vi "bucketOf.vi"(8 "error in (no error)":errorcluster, 10 "Key":string, 11 "HashMap in":refnum<class "HashMap.lvclass">) -> (0 "error out":errorcluster, 2 "Bucket Index":u32, 3 "HashMap out":refnum<class "HashMap.lvclass">)   [LabVIEW 2017, in "HashMap.lvclass"]
uses:
  <userlib>/836-Library/Data_Structures/HashMap/HashMap.lvclass
  <userlib>/836-Library/Data_Structures/Bucket/Bucket.lvclass
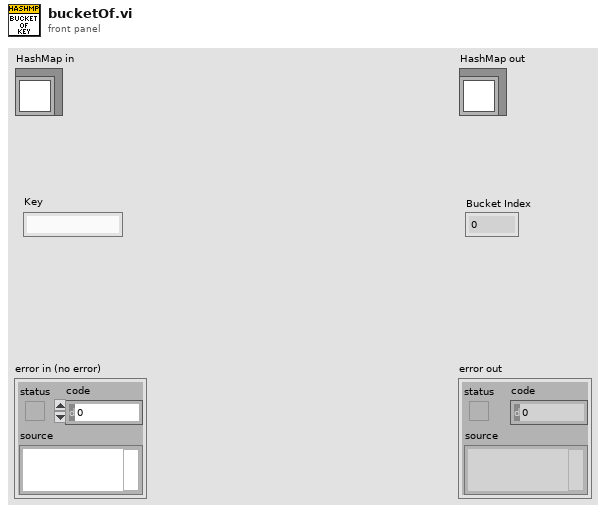
[diagram p1: front panel]
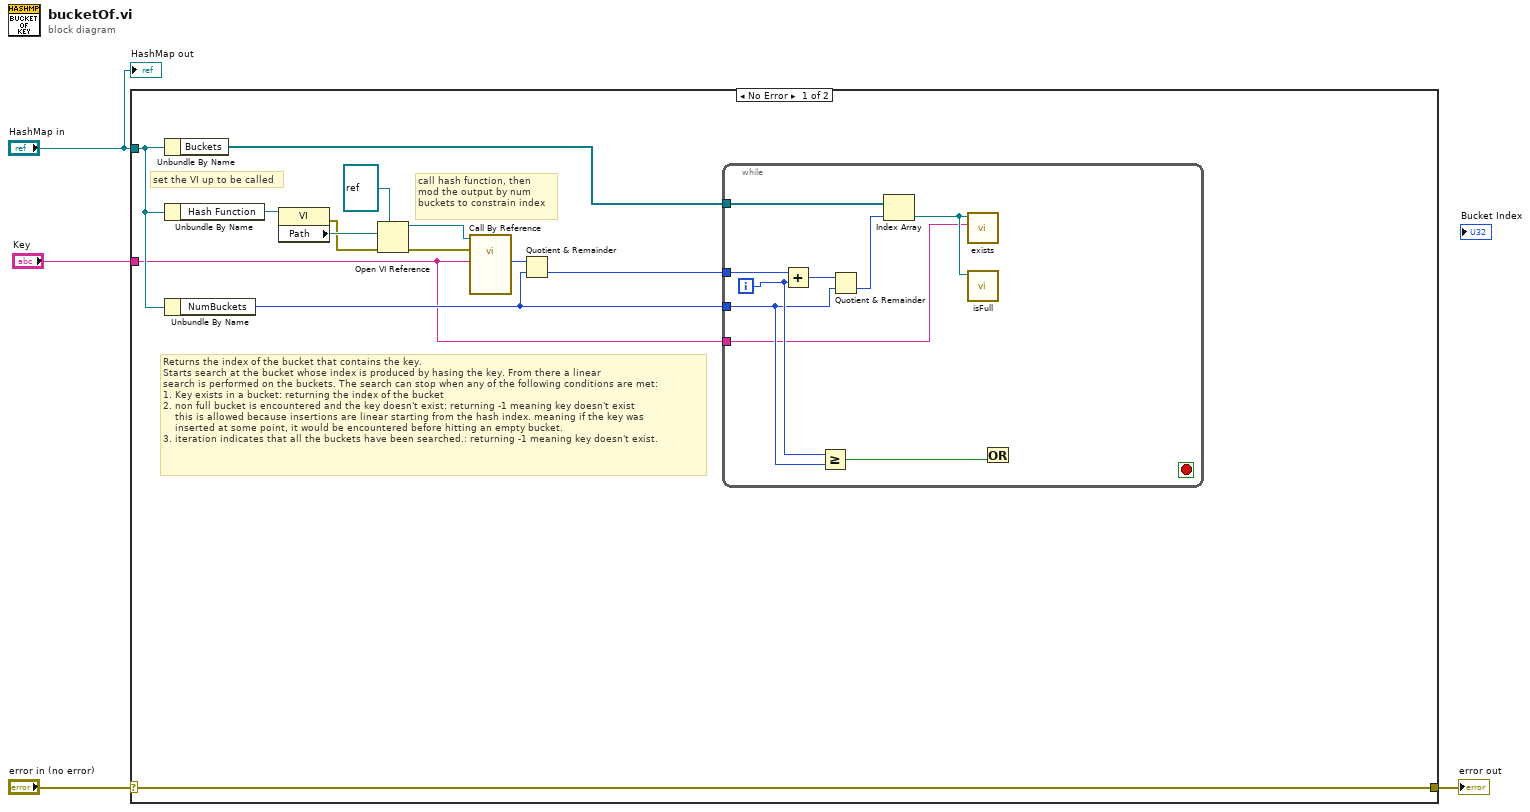
[diagram p0: block diagram]
diagram:
  n1 = case shown="No Error" "error in (no error)" {
    selector: "error in (no error)" -> [w17 w27]
    tunnel: [w17 w27] -> w3
    tunnel: "HashMap in" -> [w9 _]
    tunnel: "Key" -> [w5 _]
    frame No Error {
      # "Returns the index of the bucket that contains the key.\nStarts search at the bucket whose index is produced by hasing the key. From there a linear\nsearch is performed on the buckets. The search can stop when any of the following conditions are met:\n1. Key exists in a bucket: returning the index of the bucket\n2. non full bucket is encountered and the key doesn't exist: returning -1 meaning key doesn't exist\n    this is allowed because insertions are linear starting from the hash index. meaning if the key was\n    inserted at some point, it would be encountered before hitting an empty bucket.\n3. iteration indicates that all the buckets have been searched.: returning -1 meaning key doesn't exist."
      # "call hash function, then\nmod the output by num\nbuckets to constrain index"
      # "set the VI up to be called"
      n2 = Unbundle By Name(w9) -> ("Buckets"=w8:refnum<class "Bucket.lvclass">[])
      n3 = Unbundle By Name(w9) -> ("Hash Function"=w16:refnum<vi>)
      n4 = Unbundle By Name(w9) -> ("NumBuckets"=w6:u32)
      n5 = property class="VI"(reference=w16) -> (error out=w12:errorcluster, "Path"=w15:path)  [unwired: 1 in, 1 out]
      n6 = Open VI Reference(type specifier VI Refnum (for type only)=refnum<vi> refnum, vi path=w15, error in (no error)=w12) -> (vi reference=w13:refnum<vi>, error out=w11:errorcluster)  [unwired: 3 in]
      n7 = call-by-ref "?"(reference=w13, error in=w11, "Key"=w5) -> ("Hash"=w10:i32)  [unwired: 10 in, 2 out]
      n8 = Quotient & Remainder(x=w10, y=w6) -> (floor(x/y)=w7:u32)  [unwired: 1 out]
      n9 = while {
        tunnel: w8 -> [w24]
        tunnel: w7 -> [w26]
        tunnel: w6 -> [w21]
        tunnel: w5 -> [w18]
        i -> [w22]
        stop <- _ stop-if-true
        n10 = Add(x=w26, y=w22) -> (x+y=w25:u32)
        n11 = Greater Or Equal?(x=w22, y=w21) -> (x >= y?=w20:bool)
        n12 = Quotient & Remainder(x=w25, y=w21) -> (floor(x/y)=w23:u32)  [unwired: 1 out]
        n13 = Index Array(array=w24, index=w23) -> (element=w19:refnum<class "Bucket.lvclass">)
        n14 = call <userlib>:"exists.vi"("Key"=w18, "Bucket in"=w19) -> ()  [unwired: 7 in, 3 out]
        n15 = call <userlib>:"isFull.vi"("Bucket in"=w19) -> ()  [unwired: 8 in, 3 out]
        n16 = Or(y=w20) -> ()  [unwired: 1 in, 1 out]
      }
    }
    frame Error {
    }
  }
  "error out" <- w3
  "HashMap out" <- "HashMap in"
